vi "Default Values.vi"(7 "Type":refnum<class "TAF Proj Config.lvclass">, 8 "error in":errorcluster) -> (0 "error out":errorcluster, 3 "Lv Proj Document Type:TAF Proj Config out":refnum<class "TAF Proj Config.lvclass">)   [LabVIEW 2021, in "TAF Proj Document Type.lvlib" / "TAF Proj Config.lvclass"]
uses:
  <vilib>/Wovalab/AntiDoc/Document Type/Add-ons/LabVIEW TAF Project/TAF Proj Config/TAF Proj Config.lvclass
  <vilib>/Wovalab/AntiDoc/Document Type/Add-ons/LabVIEW TAF Project/TAF Proj Config/TAF Proj Config.lvclass/TAF Proj Config.ctl
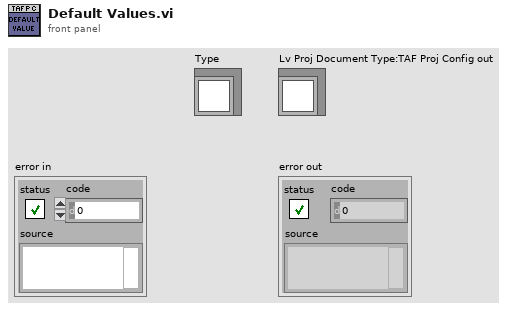
[diagram p1: front panel]
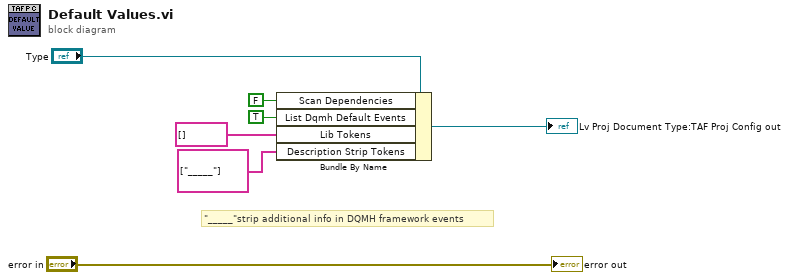
[diagram p0: block diagram]
diagram:
  # "\"_____\"strip additional info in DQMH framework events"
  n1 = Bundle By Name(cluster="Type", "Scan Dependencies"=FALSE, "List Dqmh Default Events"=TRUE, "Lib Tokens"=string[] [], "Description Strip Tokens"=string[] ["_____"] ("Lib Tokens")) -> (→"Lv Proj Document Type:TAF Proj Config out":refnum<class "TAF Proj Config.lvclass">)
  "error out" <- "error in"
